vi "close Tx.vi"(8 "error in (no error)":errorcluster, 11 "UDP Tx in":refnum<class "UDP Tx.lvclass">) -> (0 "error out":errorcluster)   [LabVIEW 2012, in "UDP Tx.lvclass"]
uses:
  UDP Tx.lvclass
  UDP Tx.lvclass/UDP Tx.ctl
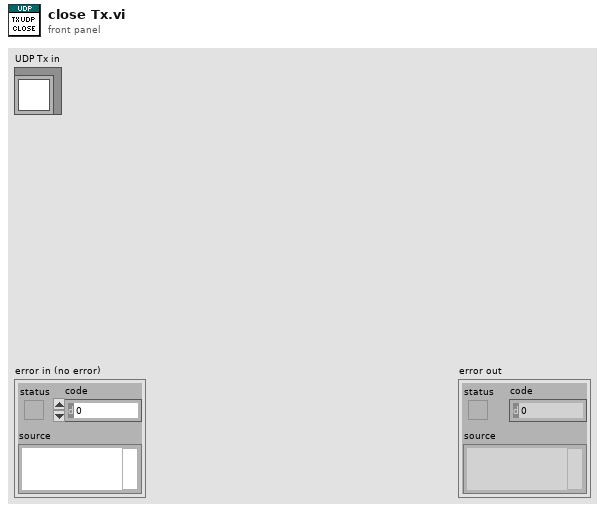
[diagram p1: front panel]
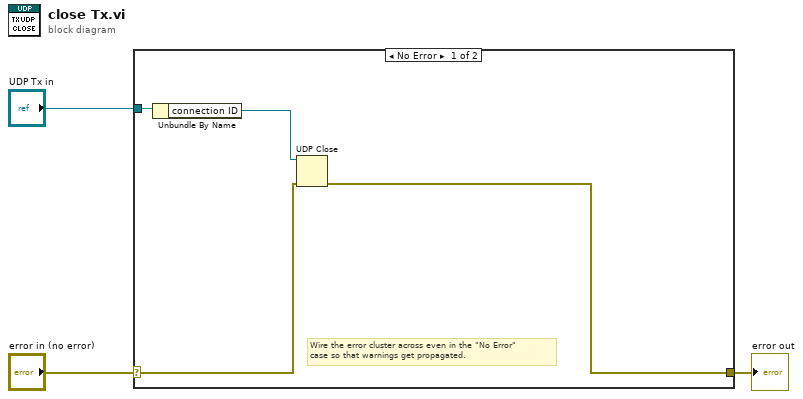
[diagram p0: block diagram]
diagram:
  n1 = case shown="No Error" "error in (no error)" {
    selector: "error in (no error)" -> [w5 w8]
    tunnel: [w4 w8] -> w2
    tunnel: "UDP Tx in" -> [w7 _]
    frame No Error {
      # "Wire the error cluster across even in the \"No Error\"\ncase so that warnings get propagated."
      n2 = Unbundle By Name(w7) -> ("connection ID"=w6:refnum<k16>)
      n3 = UDP Close(connection ID=w6, 8:w5) -> (error out=w4:errorcluster)  [unwired: 1 out]
    }
    frame Error {
    }
  }
  "error out" <- w2
